vi "Periodic Tasks.vi"(8 "error in":errorcluster) -> ()   [LabVIEW 2015]
doc: "This VI runs in parallel to other tasks. It can contain as many user-defined periodic loops as you need. These can carry out PID or other sorts of timed response."
uses:
  <vilib>/Rock Robotics/WPI/Utilities/WPI_GetSetVariantRefNum.vi
  Robot Global Data.vi
  <vilib>/Rock Robotics/Network Tables/NT Write Number.vi
  <vilib>/Rock Robotics/Network Tables/NT Read Number.vi
  <vilib>/Rock Robotics/Network Tables/NT Read Boolean.vi
  navX Library v2/navX Library v2.lvlib
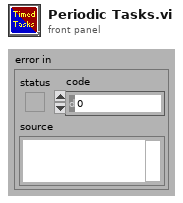
[diagram p1: front panel]
types:
  T1 = typedef "navX Library v2.lvlib/Z900_navX_DeviceTypeDef.ctl" = cluster{"Interface":cluster{"Protocol":T2, "Update Rate (4Hz-60Hz)":u8, "navX Open TypeDef":variant}, "Notify Packet":refnum<notifier>, "Loop VI Refnum":refnum<vi>, "Ready to Close Occurrence Refnum":refnum<k4>}
  T2 = typedef "navX Library v2.lvlib/Z900_navX_ProtocolTypeDef.ctl" = enum16{"SERIAL", "I2C", "SPI"}
  T3 = typedef "WPI_EncoderDevRef.ctl" = cluster{"DevStatus":errorcluster, "EncoderIndex":T4, "CounterIndex":T5, "DistancePerCount":dbl, "Decoding Type":T6}
  T4 = typedef "FPGA_EncoderIdx.ctl" = enum8{"Enc 0", "Enc 1", "Enc 2", "Enc 3", "Enc 4", "Enc 5", "Enc 6", "Enc 7", "Invalid"}
  T5 = typedef "FPGA_CounterCtrSystemIndex.ctl" = enum8{"Ctr 0", "Ctr 1", "Ctr 2", "Ctr 3", "Ctr 4", "Ctr 5", "Ctr 6", "Ctr 7", "Invalid"}
  T6 = typedef "WPI_EncoderType.ctl" = enum16{"1x", "2x", "4x"}
  T7 = cluster{"Yaw":dbl, "Roll":dbl, "Pitch":dbl, "Heading":dbl, "Fused Heading":dbl}
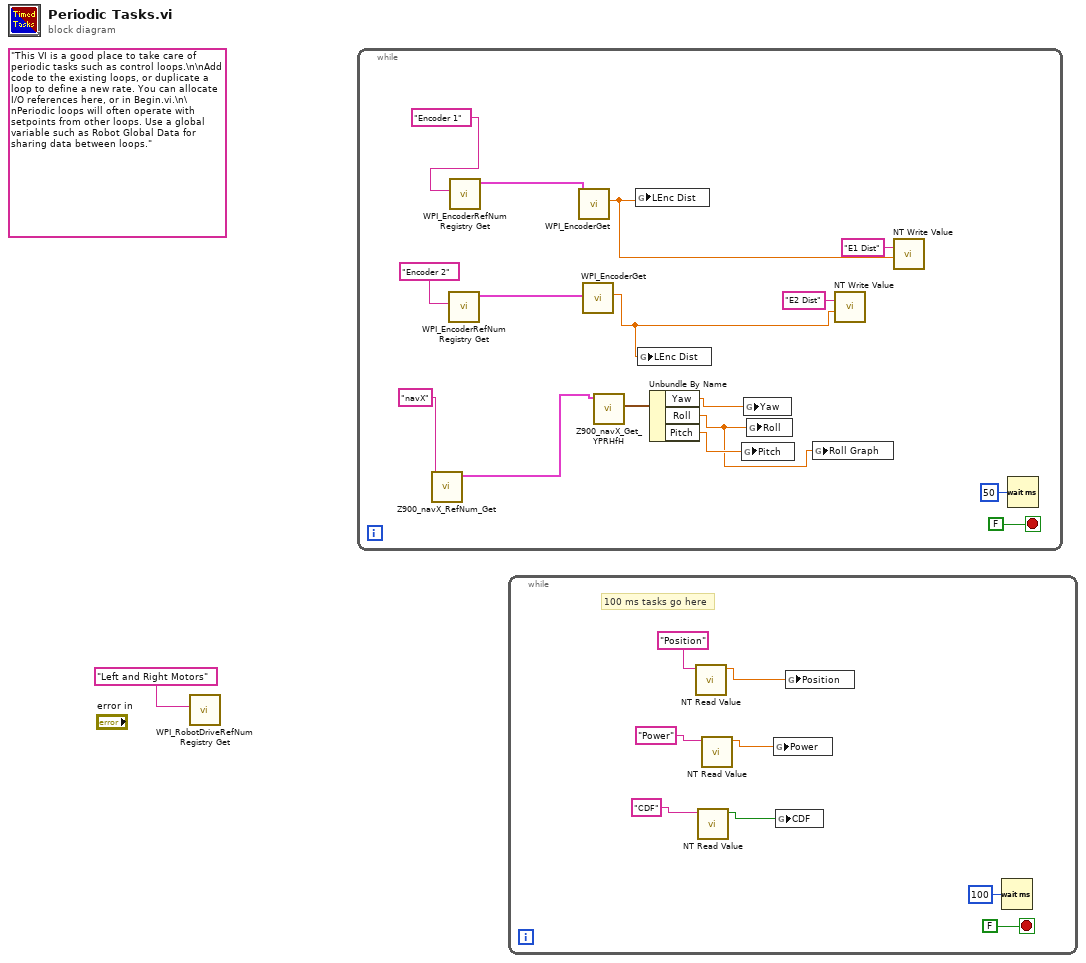
[diagram p0: block diagram]
diagram:
  (unwired) "This VI is a good place to take care of periodic tasks such as control loops.\n\nAdd code to the existing loops, or duplicate a loop to define a new rate. You can allocate I/O references here, or in Begin.vi.\n\nPeriodic loops will often operate with setpoints from other loops. Use a global variable such as Robot Global Data for sharing data between loops."
  n1 = call <vilib>:"WPI_RobotDriveRefNum Registry Get.vi"("refnum name"="Left and Right Motors") -> ()  [unwired: 1 in, 10 out]
  n2 = while {
    stop <- FALSE stop-if-true
    n3 = call "Z900_navX_RefNum_Get.vi"("refnum name"="navX") -> ("navX Device"=w4:T1)  [unwired: 9 in, 1 out]
    n4 = call <vilib>:"WPI_EncoderRefNum Registry Get.vi"("refnum name"="Encoder 2") -> ("EncoderDevRef"=w6:T3)  [unwired: 9 in, 1 out]
    n5 = call <vilib>:"WPI_EncoderRefNum Registry Get.vi"("refnum name"="Encoder 1") -> ("EncoderDevRef"=w5:T3)  [unwired: 9 in, 1 out]
    n6 = call <vilib>:"WPI_EncoderGet.vi"("EncoderDevRef"=w5) -> ("Distance"=w8:dbl)  [unwired: 5 in, 5 out]
    n7 = call <vilib>:"WPI_EncoderGet.vi"("EncoderDevRef"=w6) -> ("Distance"=w7:dbl)  [unwired: 5 in, 5 out]
    n8 = call "Z900_navX_Get_YPRHfH.vi"("navX Device"=w4) -> ("YRPHfH"=w12:T7)  [unwired: 7 in, 3 out]
    n9 = global write "Robot Global Data.vi" "LEnc Dist"(w8) -> ()
    n10 = global write "Robot Global Data.vi" "LEnc Dist"(w7) -> ()
    n11 = Unbundle By Name(w12) -> ("Yaw"=w11:dbl, "Roll"=w2:dbl, "Pitch"=w3:dbl)
    n12 = global write "Robot Global Data.vi" "Pitch"(w3) -> ()
    n13 = global write "Robot Global Data.vi" "Yaw"(w11) -> ()
    n14 = global write "Robot Global Data.vi" "Roll"(w2) -> ()
    n15 = global write "Robot Global Data.vi" "Roll Graph"(w2) -> ()
    n16 = call-poly <vilib>:"NT Write Value.vi"("Numeric"=w7, "Name"="E2 Dist") -> ()  [unwired: 9 in, 1 out]
    n17 = call-poly <vilib>:"NT Write Value.vi"("Numeric"=w8, "Name"="E1 Dist") -> ()  [unwired: 9 in, 1 out]
    n18 = Wait (ms)(milliseconds to wait=u32 50) -> ()  [unwired: 1 out]
  }
  n19 = while {
    stop <- FALSE stop-if-true
    # "100 ms tasks go here"
    n20 = call-poly <vilib>:"NT Read Value.vi"("Name"="Position") -> ("Numeric"=w23:dbl)  [unwired: 9 in, 1 out]
    n21 = call-poly <vilib>:"NT Read Value.vi"("Name"="CDF") -> ("Boolean"=w19:bool)  [unwired: 9 in, 1 out]
    n22 = call-poly <vilib>:"NT Read Value.vi"("Name"="Power") -> ("Numeric"=w21:dbl)  [unwired: 9 in, 1 out]
    n23 = global write "Robot Global Data.vi" "Power"(w21) -> ()
    n24 = global write "Robot Global Data.vi" "CDF"(w19) -> ()
    n25 = global write "Robot Global Data.vi" "Position"(w23) -> ()
    n26 = Wait (ms)(milliseconds to wait=u32 100) -> ()  [unwired: 1 out]
  }
